vi "RFSA Power vs Time (Zero-Span).vi"(4 "Single Acquisition?":bool, 5 "Samples to Read per Block":i32=1000, 6 "IQ Rate (S/s)":dbl=1000000.0 format="%#.3p", 7 "Resource Name":refnum<k15>="RFSA", 8 "error in":errorcluster {"code" format="%.0x"}, 9 "Carrier Frequency (Hz)":dbl=1000000000.0 format="%#.3p", 10 "Reference Level (dBm)":dbl format="%.2f", 11 "anlaysis queue":refnum<queue>) -> (0 "error out":errorcluster {"code" format="%.0x"})   [LabVIEW 2021]
doc: "Demonstrates how to acquire I/Q data using the RF vector signal analyzer. The example shows how to configure NI-RFSA for continuous I/Q acquisition, how to set the carrier frequency and the I/Q rate, and how to fetch I/Q data. The dBm calculation is applied to I/Q magnitude to produce signal power and display it on the graph."
uses:
  <instrlib>/niRFSA/niRFSA.llb/niRFSA Fetch IQ (Complex WDT 1Rec 1Chan).vi
  Messaging/Waveform Queue Data.ctl
  Messaging/Data Processing.ctl
panel:
  out "Seconds per Acquisition":dbl format="%#_4psec"
  out "Bytes per Second":dbl format="%#_5pB/sec"
  out "Seconds per Iteration":dbl format="%#_4psec"
  out "Bytes per Acquisition":i32 format="%.1pB"
  out "IQ Data":cluster{"X":dbl, "Y":dbl}[](graph)
  out "Mean Power":dbl
  in  "Stop":bool
  in  "Power Scaling":bool
  # "RMS"
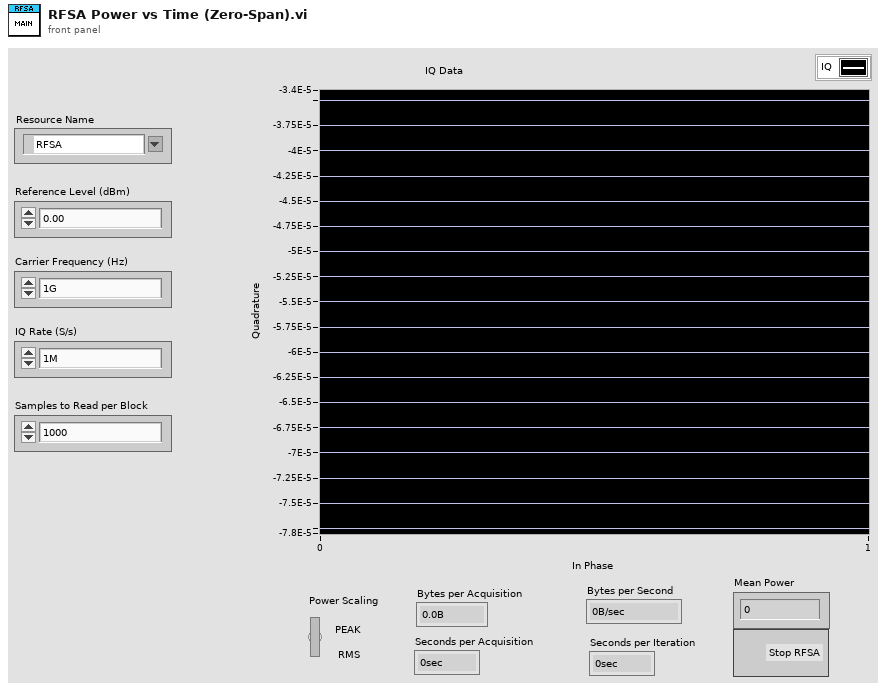
[diagram p1: front panel]
types:
  T1 = typedef "Waveform Queue Data.ctl" = cluster{"wfm dat":waveform(cdb), "msg":T2, "pwr sptm":cluster{"f0":dbl, "df":dbl, "magnitude":dbl[]}}
  T2 = typedef "Data Processing.ctl" = enum16{"Analyze", "Stream to Disk", "Analyze and Plot", "Analyze and Stream to Disk", "Analyze, Plot, and Stream to Disk", "Plot", "Exit"}
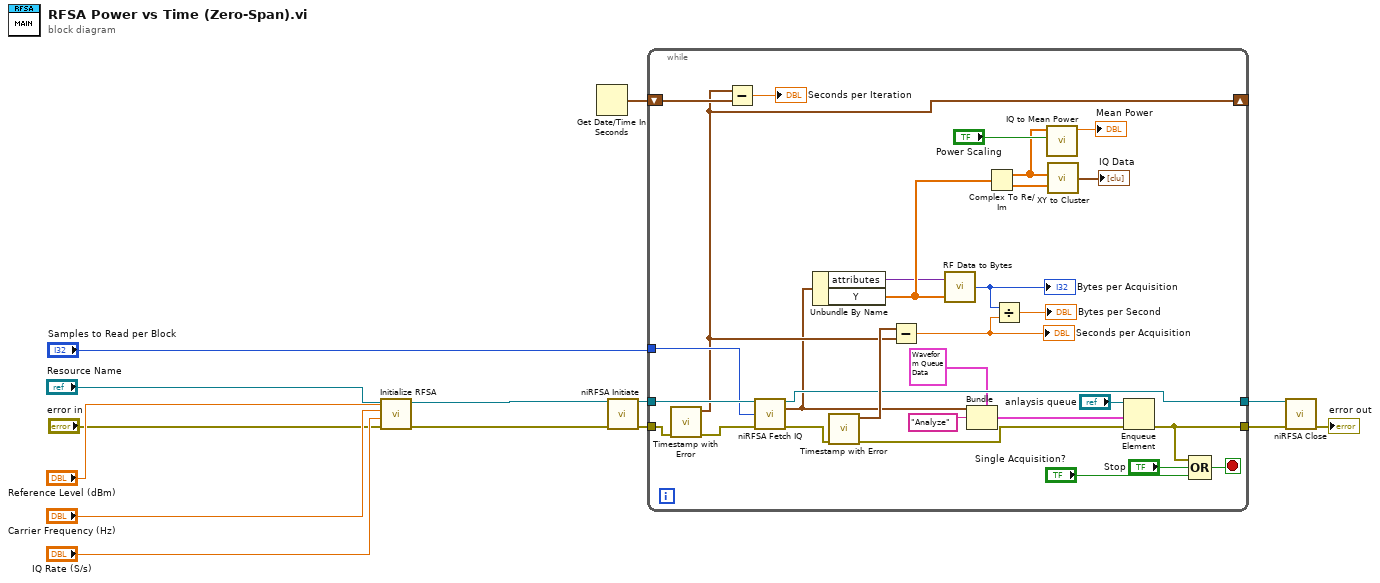
[diagram p0: block diagram]
diagram:
  n1 = call "Initialize RFSA.vi"("Reference Level"="Reference Level (dBm)", "error in (no error)"="error in", "IQ Rate"="IQ Rate (S/s)", "Carrier Frequency"="Carrier Frequency (Hz)", "RFSA Reference In"="Resource Name") -> ("error out"=w5:errorcluster, "RFSA Reference Out"=w4:refnum<k15>)  [unwired: 5 in]
  n2 = Get Date/Time In Seconds() -> (seconds since 1Jan1904=w6:timestamp)
  n3 = call <instrlib>:"niRFSA Initiate.vi"("instrument handle"=w4, "error in"=w5) -> ("instrument handle out"=w14:refnum<k15>, "error out"=w8:errorcluster)  [unwired: 12 in]
  n4 = while {
    tunnel: [w34] -> w13
    tunnel: w14 -> [w42]
    tunnel: w8 -> [w40]
    shift-right: [w30] -> _
    shift-left: w6 -> [w44]
    tunnel: "Samples to Read per Block" -> [w41]
    tunnel: [w17] -> w1
    stop <- w18 stop-if-true
    n5 = call "Timestamp with Error.vi"("error in (no error)"=w40) -> ("error out"=w39:errorcluster, "Timestamp"=w30:timestamp)  [unwired: 9 in]
    n6 = Subtract(x=w30, y=w44) -> (x-y=→"Seconds per Iteration":dbl)
    n7 = call-poly <instrlib>:"niRFSA Fetch IQ.vi"("instrument handle"=w42, "samples to read (-1)"=w41, "error in"=w39) -> ("instrument handle out"=w34:refnum<k15>, "data"=w26:waveform(cdb), "error out"=w38:errorcluster)  [unwired: 10 in]
    n8 = Unbundle By Name(w26) -> ("attributes"=w19:variant, "Y"=w23:cdb[])
    n9 = call "Timestamp with Error.vi"("error in (no error)"=w38) -> ("error out"=w29:errorcluster, "Timestamp"=w35:timestamp)  [unwired: 9 in]
    n10 = Subtract(x=w35, y=w30) -> (x-y=w37:dbl)
    "Seconds per Acquisition" <- w37
    n11 = call "RF Data to Bytes.vi"("Y"=w23, "attributes"=w19) -> ("Bytes"=w20:i32)
    "Bytes per Acquisition" <- w20
    n12 = Bundle(cluster=T1 {"wfm dat"={"t0"=timestamp(0 s since 1904-01-01), "dt"=0.0, "Y"=[]}, "msg"=enum."Analyze", "pwr sptm"={"f0"=0.0, "df"=0.0, "magnitude"=[]}} ("element"), "wfm dat"=w26, "msg"="Analyze") -> (w24:T1)  [unwired: 1 in]
    n13 = Complex To Re/Im(x + iy=w23) -> (x=w22:dbl[], y=w21:dbl[])
    n14 = Divide(x=w20, y=w37) -> (x/y=→"Bytes per Second":dbl)
    n15 = call "IQ to Mean Power.vi"("Power Scaling"="Power Scaling", "IQ Data"=w22) -> ("Mean Power"=→"Mean Power":dbl)  [unwired: 9 in]
    n16 = call "XY to Cluster.vi"("X Data"=w21, "Y Data"=w22) -> ("XY Cluster Array"=→"IQ Data":cluster{"Numeric":dbl, "Numeric":dbl}[])
    n17 = Enqueue Element(queue="anlaysis queue", element=w24, error in (no error)=w29) -> (error out=w17:errorcluster)  [unwired: 1 in, 2 out]
    n18 = Compound Arithmetic op=OR(w17, "Stop", "Single Acquisition?") -> (w18:bool)
  }
  n19 = call <instrlib>:"niRFSA Close.vi"("instrument handle"=w13, "error in"=w1) -> ("error out"=→"error out":errorcluster)  [unwired: 13 in]
